vi "Select Arbitrary Waveform.vi"(6 "Arbitrary Waveform Name (\"wave1\")":string="wave1", 7 "Channel (1:Channel 1)":i32(ring)=1 items=["Channel 1"=1, "Channel 2"=2], 8 "error in (no error)":errorcluster, 9 "Arbitrary Waveform Location (2)":i32=2, 10 "Select Waveform (0:Location)":u16(ring) items=["Location", "Name"], 11 "VISA resource name":refnum<visa-resource-name>) -> (0 "error out":errorcluster, 3 "VISA resource name out":refnum<visa-resource-name>)   [LabVIEW 2015, in "SDG X Series.lvlib"]
doc: "Selects an arbitrary waveform to output from the memory. Choose from built-in or user-defined arbitrary waveforms."
uses:
  <instrlib>/SDG X Series/SDG X Series.lvlib
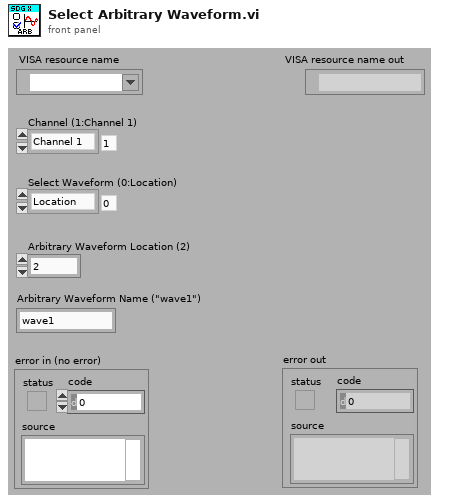
[diagram p1: front panel]
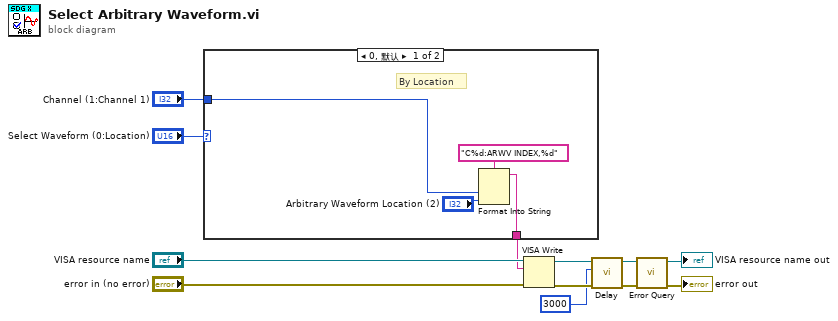
[diagram p0: block diagram]
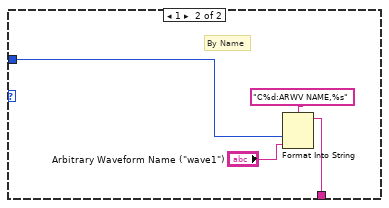
[diagram p2: hidden frame]
diagram:
  n1 = case shown="0, 默认" "Select Waveform (0:Location)" {
    tunnel: "Channel (1:Channel 1)" -> [w15 w19]
    tunnel: [w14 w17] -> w10
    frame 0, Default {
      # "By Location"
      n2 = Format Into String(format string="C%d:ARWV INDEX,%d", w15, "Arbitrary Waveform Location (2)") -> (resulting string=w14:string)  [unwired: 2 in, 1 out]
    }
    frame 1 {
      # "By Name"
      n3 = Format Into String(format string="C%d:ARWV NAME,%s", w19, "Arbitrary Waveform Name (\"wave1\")") -> (resulting string=w17:string)  [unwired: 2 in, 1 out]
    }
  }
  n4 = VISA Write(VISA resource name="VISA resource name", write buffer=w10, error in (no error)="error in (no error)") -> (VISA resource name out=w7:refnum<visa-resource-name>, error out=w6:errorcluster)  [unwired: 1 out]
  n5 = call <instrlib>:"Delay.vi"("error in (no error)"=w6, "Delay Time (10)"=u32 3000, "VISA resource name"=w7) -> ("error out"=w4:errorcluster, "VISA resource name out"=w3:refnum<visa-resource-name>)  [unwired: 7 in]
  n6 = call <instrlib>:"Error Query.vi"("error in (no error)"=w4, "VISA resource name"=w3) -> ("error out"=→"error out":errorcluster, "VISA resource name out"=→"VISA resource name out":refnum<visa-resource-name>)  [unwired: 6 in, 2 out]
